vi "Read Key (Variant).vi"(5 "format string (%;%f)":string="%f", 7 "section":string, 8 "error in (no error)":errorcluster, 9 "type":variant, 10 "key (optional)":string, 11 "refnum":T1) -> (0 "error out":errorcluster, 1 "key-value":variant, 2 "found?":bool, 3 "refnum out":T1)   [LabVIEW 2020, in "openg_variant_configuration_file.lvlib"]
doc: "Reads a value associated with key in a specified section of the configuration data identified by refnum. If \"key\" input is not specified, the name of the variant object is used as the key. the \"found?\" output will be TRUE for compount objects (clusters) only if all elements (recursively) are found.\n\nFor example a Boolean named \"Enable\" with a value of TRUE would correspond to the key-value pair:\n\nEnable=TRUE\n\nNote: Special characters in section and key names will be escape-coded. These include the following: \\00-\\1F (non-printable chars); \"[\", \"]\", and \"=\" (INI syntax elements); \\FE (\"þ\") and \\FF (\"ÿ\") (legacy bracket encoding); Additionally, the escape character, \"\\\", will be escaped as \"\\\\\"."
uses:
  openg_variant_configuration_file.lvlib
  <vilib>/Utility/config.llb/Config Data RefNum.ctl
  <vilib>/Utility/config.llb/Read Key (I32).vi
  <vilib>/Utility/config.llb/Read Key (U32).vi
  <vilib>/Utility/config.llb/Read Key (Double).vi
  <vilib>/Utility/config.llb/Read Key (String).vi
  <vilib>/Utility/config.llb/Read Key (Boolean).vi
  <vilib>/Utility/config.llb/Read Key (Path).vi
  <vilib>/Utility/config.llb/NI_LVConfig.lvlib
  <userlib>/_OpenG.lib/lvdata/lvdata.llb/openg_variant.lvlib
panel:
  in  "Ref for recursive call":refnum<vi>
  # "Read Key (Variant).vi\n\nReads a variant key-value from INI file.\n\nPlease visit http://www.OpenG.org to learn about the\nOpen Source LabVIEW software movement.\n\nNOTICE -- YOU MUST LEAVE THIS NOTICE IN PLACE.  PER THE TERMS OF THE LICENSE BELOW, YOU MAY SUBLICENSE THIS SOFTWARE \nIN ANY WAY THAT DOES NOT CONFLICT WITH THIS LICENSE.\n\n### BSD License (http://www.opensource.org/licenses/bsd-license.php) Begin ###\n \nCopyright (c) 2002, Jean-Pierre Drolet <drolet_jp@hotmail.com>\nCopyright (c) 2002-2006, Jim Kring <jim@jimkring.com>\n\nAll rights reserved.\n\nRedistribution and use in source and binary forms, with or without modification, are permitted provided that the following conditions are met:\n\n    * Redistributions of source code must retain the above copyright notice, this list of conditions and the following disclaimer.\n    * Redistributions in binary form must reproduce the above copyright notice, this list of conditions and the following disclaimer in the \n       documentation and/or other materials provided with the distribution.\n    * Neither the name of SciWare, James Kring, Inc., nor the names of its contributors may be used to endorse or promote products derived \n       from this software without specific prior written permission.\n\nTHIS SOFTWARE IS PROVIDED BY THE COPYRIGHT HOLDERS AND CONTRIBUTORS \"AS IS\" AND ANY EXPRESS OR IMPLIED WARRANTIES, \nINCLUDING, BUT NOT LIMITED TO, THE IMPLIED WARRANTIES OF MERCHANTABILITY AND FITNESS FOR A PARTICULAR PURPOSE ARE \nDISCLAIMED. IN NO EVENT SHALL THE COPYRIGHT OWNER OR CONTRIBUTORS BE LIABLE FOR ANY DIRECT, INDIRECT, INCIDENTAL,\n SPECIAL, EXEMPLARY, OR CONSEQUENTIAL DAMAGES (INCLUDING, BUT NOT LIMITED TO, PROCUREMENT OF SUBSTITUTE GOODS OR \nSERVICES; LOSS OF USE, DATA, OR PROFITS; OR BUSINESS INTERRUPTION) HOWEVER CAUSED AND ON ANY THEORY OF LIABILITY, \nWHETHER IN CONTRACT, STRICT LIABILITY, OR TORT (INCLUDING NEGLIGENCE OR OTHERWISE) ARISING IN ANY WAY OUT OF THE USE \nOF THIS SOFTWARE, EVEN IF ADVISED OF THE POSSIBILITY OF SUCH DAMAGE.\n\n### BSD License End ###"
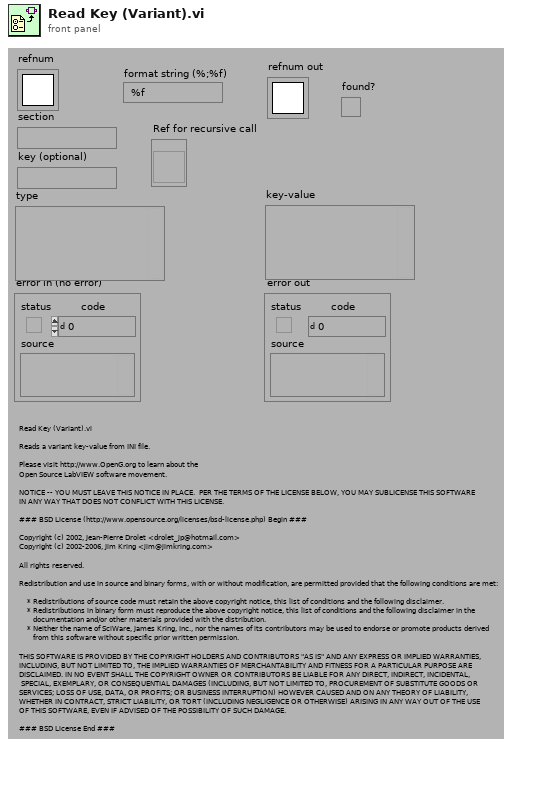
[diagram p1: front panel]
types:
  T1 = typedef "NI_LVConfig.lvlib/Config Data RefNum.ctl" = refnum<k1>
  T2 = typedef "openg_variant.lvlib/Type Descriptor Enumeration__ogtk.ctl" = enum8{"<Null>", "I8", "I16", "I32", "I64", "U8", "U16", "U32", "U64", "SGL", "DBL", "EXT", "CSG", "CDB", "CXT", "0x0F", "0x10", "0x11", "0x12", "0x13", "0x14", "Enum U8", "Enum U16", "Enum U32", "Enum U64", "SGL PQ", "DBL PQ", "EXT PQ", "CSG PQ", "CDB PQ", "CXT PQ", "0x1F", "0x20", "Boolean", "0x22", "0x23", "0x24", "0x25", "0x26", "0x27", "0x28", "0x29", "0x2A", "0x2B", "0x2C", "0x2D", "0x2E", "0x2F", "String", "0x31", "Path", "Pict", "0x34", "0x35", "0x36", "DAQ", "0x38", "0x39", "0x3A", "0x3B", "0x3C", "0x3D", "0x3E", "0x3F", "Array", "0x41", "0x42", "0x43", "0x44", "0x45", "0x46", "0x47", "0x48", "0x49", "0x4A", "0x4B", "0x4C", "0x4D", "0x4E", "0x4F", "Cluster", "0x51", "0x52", "Variant", "Waveform", "0x55", "0x56", "0x57", "0x58", "0x59", "0x5A", "0x5B", "0x5C", "0x5D", "0x5E", "Fixed Point", "0x60", "0x61", "0x62", "0x63", "0x64", "0x65", "0x66", "0x67", "0x68", "0x69", "0x6A", "0x6B", "0x6C", "0x6D", "0x6E", "0x6F", "Refnum", "0x71", "0x72", "Set Collection", "Map Collection"}
  T3 = typedef "openg_variant.lvlib/Type Descriptor__ogtk.ctl" = i16[]
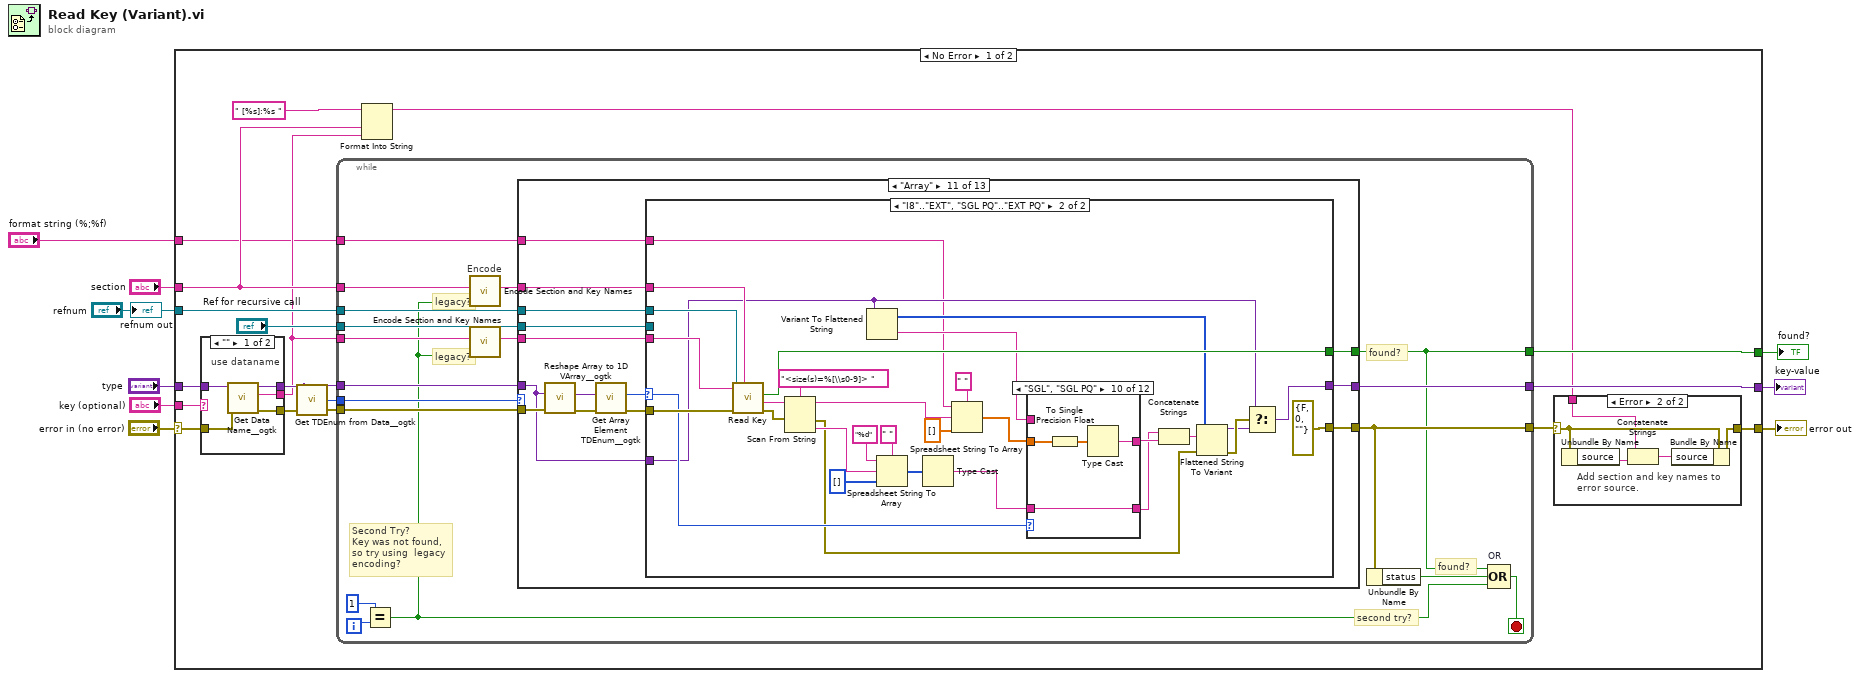
[diagram p0: block diagram]
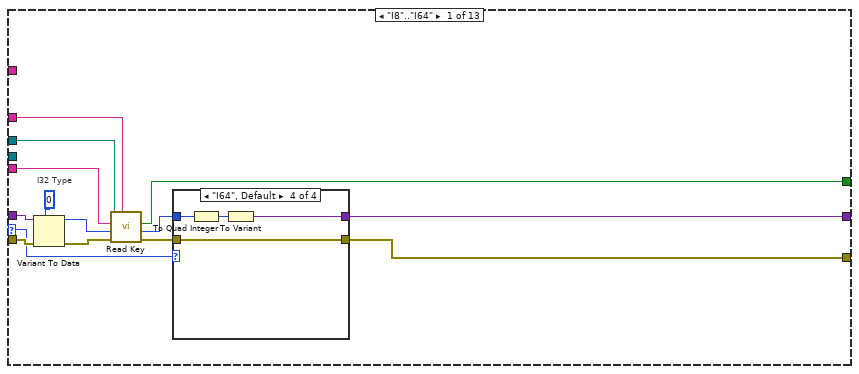
[diagram p2: hidden frame]
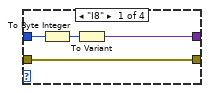
[diagram p3: hidden frame]
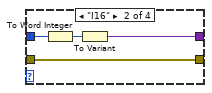
[diagram p4: hidden frame]
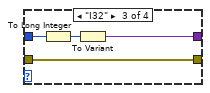
[diagram p5: hidden frame]
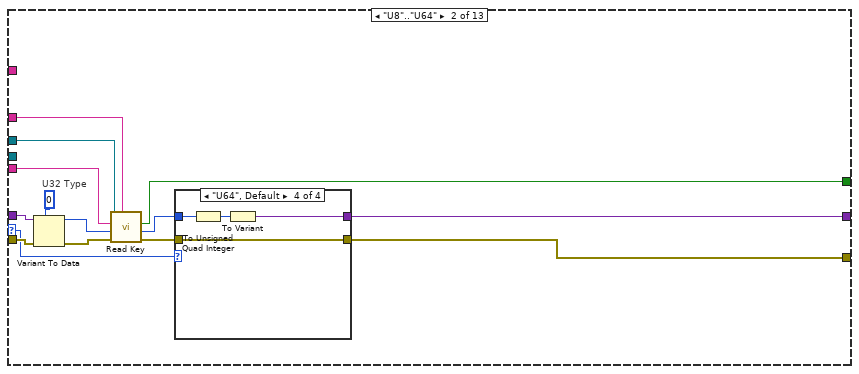
[diagram p6: hidden frame]
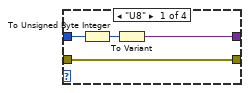
[diagram p7: hidden frame]
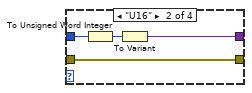
[diagram p8: hidden frame]
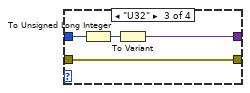
[diagram p9: hidden frame]
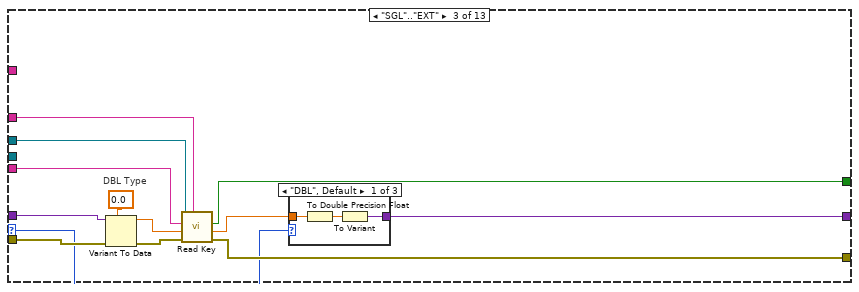
[diagram p10: hidden frame]
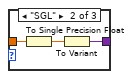
[diagram p11: hidden frame]
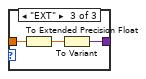
[diagram p12: hidden frame]
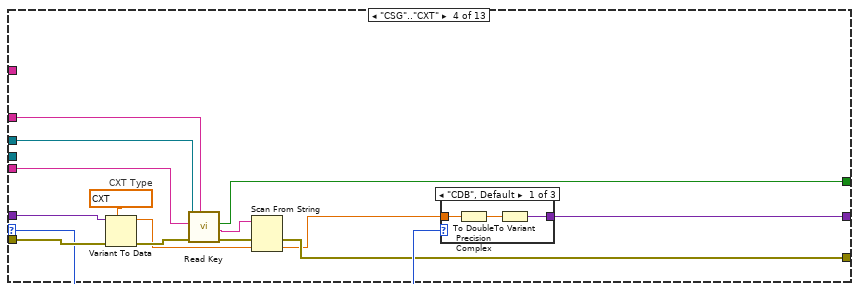
[diagram p13: hidden frame]
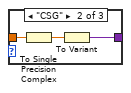
[diagram p14: hidden frame]
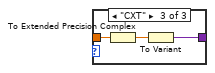
[diagram p15: hidden frame]
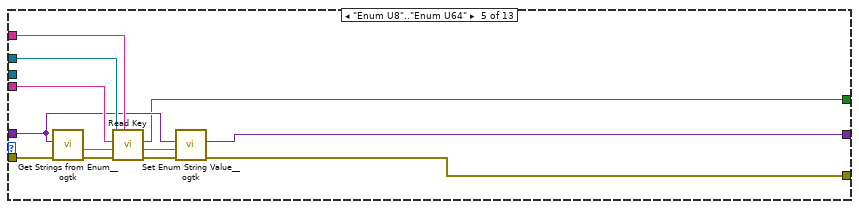
[diagram p16: hidden frame]
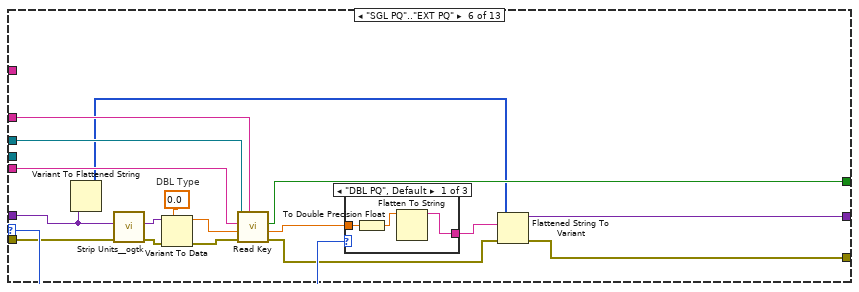
[diagram p17: hidden frame]
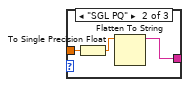
[diagram p18: hidden frame]
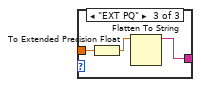
[diagram p19: hidden frame]
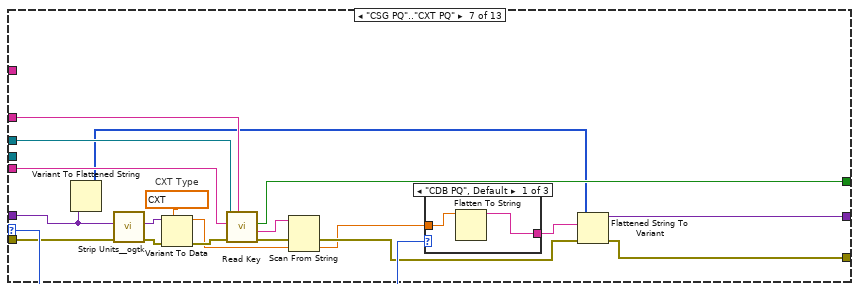
[diagram p20: hidden frame]
diagram:
  n1 = case shown="No Error" "error in (no error)" {
    selector: "error in (no error)" -> [w21 w480]
    tunnel: "refnum" -> [w25 _]
    tunnel: [w15 w480] -> w9
    tunnel: "type" -> [w23 _]
    tunnel: "key (optional)" -> [w22 _]
    tunnel: "section" -> [w12 _]
    tunnel: [w24 variant ("Variant")] -> w4
    tunnel: [w18 FALSE ("found?")] -> w2
    tunnel: "format string (%;%f)" -> [w10 _]
    frame No Error {
      n2 = case shown="\"\"" w22 {
        selector: w22 -> [_ w477]
        tunnel: [w474 w477] -> w11
        tunnel: w23 -> [w471 w475]
        tunnel: w21 -> [w473 w476]
        tunnel: [w472 w476] -> w20
        tunnel: [w470 w475] -> w19
        frame "" {
          # "use dataname"
          n3 = call <userlib>:"Get Data Name__ogtk.vi"("error in (no error)"=w473, "Data"=w471) -> ("error out"=w472:errorcluster, "Data Name"=w474:string, "Data dup"=w470:variant)  [unwired: 7 in]
        }
        frame Default {
          # "use optional\nkey"
        }
      }
      n4 = call <userlib>:"Get TDEnum from Data__ogtk.vi"("Data"=w19) -> ("Type Descriptor Enumeration"=w26:T2)  [unwired: 4 in]
      n5 = while {
        tunnel: w26 -> [w44]
        tunnel: w25 -> [w43]
        tunnel: [w42] -> w24
        tunnel: w20 -> [w41]
        tunnel: w19 -> [w40]
        tunnel: [w32] -> w18
        tunnel: "Ref for recursive call" -> [w39]
        tunnel: [w34] -> w16
        tunnel: w12 -> [w37]
        tunnel: w11 -> [w36]
        tunnel: w10 -> [w27]
        i -> [w31]
        stop <- w29 stop-if-true
        # "found?"
        # "found?"
        # "second try?"
        # "legacy?"
        # "legacy?"
        # "Second Try?\nKey was not found, so try using  legacy encoding?"
        # "Encode"
        n6 = Equal?(x=1, y=w31) -> (x = y?=w28:bool)
        n7 = call "Encode Section and Key Names.vi"("use legacy encoding scheme? (FALSE)"=w28, "string"=w37) -> ("encoded string"=w38:string)  [unwired: 9 in]
        n8 = call "Encode Section and Key Names.vi"("use legacy encoding scheme? (FALSE)"=w28, "string"=w36) -> ("encoded string"=w35:string)  [unwired: 9 in]
        n9 = case shown="\"Array\"" w44 {
          selector: w44 -> [w47 w77 w105 w132 _ w172 w203 _ _ _ _ _ _]
          tunnel: w40 -> [w57 w87 w116 w140 w153 w165 w197 w228 w240 w252 w256 w411 w460]
          tunnel: w43 -> [w56 w86 w115 w139 w162 w179 w208 w227 w239 w251 w263 w425 w463]
          tunnel: [w46 w75 w113 w130 w155 w167 w199 w225 w237 w249 w260 w414 w454] -> w34
          tunnel: w41 -> [w54 w84 w112 w137 w159 w171 w202 w224 w236 w248 w266 w413 w456]
          tunnel: w35 -> [w53 w83 w111 w136 w161 w177 w206 w223 w235 w247 w257 w423 w462]
          tunnel: w38 -> [w52 w82 w110 w135 w160 w176 w205 w222 w234 w246 w258 w424 w461]
          tunnel: [w45 w79 w107 w134 w152 w163 w195 w219 w233 w243 w261 w415 w457] -> w42
          tunnel: [w50 w78 w106 w133 w151 w173 w204 w218 w230 w242 w259 w419 w452] -> w32
          tunnel: w39 -> [_ _ _ _ _ _ _ _ _ _ w262 w418 _]
          tunnel: w27 -> [_ _ _ _ _ _ _ _ _ _ w254 w408 _]
          frame "I8".."I64" {
            # "I32 Type"
            n10 = Variant To Data(error in=w54, type=0, Variant=w57) -> (data=w51:i32, error out=w55:errorcluster)
            n11 = call-poly <vilib>:"Read Key.vi"("section"=w52, "error in (no error)"=w55, "default value"=w51, "key"=w53, "refnum"=w56) -> ("error out"=w49:errorcluster, "value"=w48:i32, "found?"=w50:bool)  [unwired: 3 in, 1 out]
            n12 = case shown="\"I64\", Default" w47 {
              tunnel: w48 -> [w62 w66 w70 w74]
              tunnel: [w61 w65 w69 w73] -> w45
              tunnel: w49 -> [w59 w63 w67 w71]
              tunnel: [w59 w63 w67 w71] -> w46
              frame "I8" {
                n13 = To Byte Integer(number=w62) -> (8bit integer=w60:i8)
                n14 = To Variant(anything=w60) -> (Variant=w61:variant)
              }
              frame "I16" {
                n15 = To Word Integer(number=w66) -> (16bit integer=w64:i16)
                n16 = To Variant(anything=w64) -> (Variant=w65:variant)
              }
              frame "I32" {
                n17 = To Long Integer(number=w70) -> (32bit integer=w68:i32)
                n18 = To Variant(anything=w68) -> (Variant=w69:variant)
              }
              frame "I64", Default {
                n19 = To Quad Integer(1:w74) -> (0:w72:i64)
                n20 = To Variant(anything=w72) -> (Variant=w73:variant)
              }
            }
          }
          frame "U8".."U64" {
            # "U32 Type"
            n21 = Variant To Data(error in=w84, type=u32 0, Variant=w87) -> (data=w81:u32, error out=w85:errorcluster)
            n22 = call-poly <vilib>:"Read Key.vi"("section"=w82, "error in (no error)"=w85, "default value"=w81, "key"=w83, "refnum"=w86) -> ("error out"=w76:errorcluster, "value"=w80:u32, "found?"=w78:bool)  [unwired: 3 in, 1 out]
            n23 = case shown="\"U64\", Default" w77 {
              tunnel: w80 -> [w92 w96 w100 w104]
              tunnel: [w91 w95 w99 w103] -> w79
              tunnel: w76 -> [w89 w93 w97 w101]
              tunnel: [w89 w93 w97 w101] -> w75
              frame "U8" {
                n24 = To Unsigned Byte Integer(number=w92) -> (unsigned 8bit integer=w90:u8)
                n25 = To Variant(anything=w90) -> (Variant=w91:variant)
              }
              frame "U16" {
                n26 = To Unsigned Word Integer(number=w96) -> (unsigned 16bit integer=w94:u16)
                n27 = To Variant(anything=w94) -> (Variant=w95:variant)
              }
              frame "U32" {
                n28 = To Unsigned Long Integer(number=w100) -> (unsigned 32bit integer=w98:u32)
                n29 = To Variant(anything=w98) -> (Variant=w99:variant)
              }
              frame "U64", Default {
                n30 = To Unsigned Quad Integer(1:w104) -> (0:w102:u64)
                n31 = To Variant(anything=w102) -> (Variant=w103:variant)
              }
            }
          }
          frame "SGL".."EXT" {
            # "DBL Type"
            n32 = Variant To Data(error in=w112, type=0.0, Variant=w116) -> (data=w109:dbl, error out=w114:errorcluster)
            n33 = call-poly <vilib>:"Read Key.vi"("section"=w110, "error in (no error)"=w114, "default value"=w109, "key"=w111, "refnum"=w115) -> ("error out"=w113:errorcluster, "value"=w108:dbl, "found?"=w106:bool)  [unwired: 3 in, 1 out]
            n34 = case shown="\"DBL\", Default" w105 {
              tunnel: w108 -> [w120 w123 w126]
              tunnel: [w119 w122 w125] -> w107
              frame "DBL", Default {
                n35 = To Double Precision Float(number=w120) -> (double precision float=w118:dbl)
                n36 = To Variant(anything=w118) -> (Variant=w119:variant)
              }
              frame "SGL" {
                n37 = To Single Precision Float(number=w123) -> (single precision float=w121:sgl)
                n38 = To Variant(anything=w121) -> (Variant=w122:variant)
              }
              frame "EXT" {
                n39 = To Extended Precision Float(1:w126) -> (0:w124:ext)
                n40 = To Variant(anything=w124) -> (Variant=w125:variant)
              }
            }
          }
          frame "CSG".."CXT" {
            # "CXT Type"
            n41 = Variant To Data(error in=w137, type=cxt 0.0+0.0i, Variant=w140) -> (data=w128:cxt, error out=w138:errorcluster)
            n42 = call-poly <vilib>:"Read Key.vi"("section"=w135, "error in (no error)"=w138, "key"=w136, "refnum"=w139) -> ("error out"=w131:errorcluster, "value"=w129:string, "found?"=w133:bool)  [unwired: 4 in, 1 out]
            n43 = Scan From String(input string=w129, error in=w131, default 1=w128) -> (error out=w130:errorcluster, output 1=w127:cxt)  [unwired: 2 in, 2 out]
            n44 = case shown="\"CDB\", Default" w132 {
              tunnel: w127 -> [w144 w147 w150]
              tunnel: [w143 w146 w149] -> w134
              frame "CDB", Default {
                n45 = To Double Precision Complex(1:w144) -> (0:w142:cdb)
                n46 = To Variant(anything=w142) -> (Variant=w143:variant)
              }
              frame "CSG" {
                n47 = To Single Precision Complex(1:w147) -> (0:w145:csg)
                n48 = To Variant(anything=w145) -> (Variant=w146:variant)
              }
              frame "CXT" {
                n49 = To Extended Precision Complex(1:w150) -> (0:w148:cxt)
                n50 = To Variant(anything=w148) -> (Variant=w149:variant)
              }
            }
          }
          frame "Enum U8".."Enum U64" {
            n51 = call <userlib>:"Get Strings from Enum__ogtk.vi"("error in (no error)"=w159, "Enum"=w153) -> ("error out"=w158:errorcluster, "String Value"=w157:string)  [unwired: 6 in, 2 out]
            n52 = call-poly <vilib>:"Read Key.vi"("section"=w160, "error in (no error)"=w158, "default value"=w157, "key"=w161, "refnum"=w162) -> ("error out"=w156:errorcluster, "value"=w154:string, "found?"=w151:bool)  [unwired: 3 in, 1 out]
            n53 = call <userlib>:"Set Enum String Value__ogtk.vi"("error in (no error)"=w156, "String Value"=w154, "Default Enum Value"=w153) -> ("error out"=w155:errorcluster, "Enum"=w152:variant)  [unwired: 7 in]
          }
          frame "SGL PQ".."EXT PQ" {
            # "DBL Type"
            n54 = Variant To Flattened String(Variant=w165) -> (1:w164:i16[])  [unwired: 1 out]
            n55 = call <userlib>:"Strip Units__ogtk.vi"("error in (no error)"=w171, "Number or 1D array with units"=w165) -> ("error out"=w169:errorcluster, "Pure Number(s) (base units)"=w170:variant)  [unwired: 8 in]
            n56 = Variant To Data(error in=w169, type=0.0, Variant=w170) -> (data=w175:dbl, error out=w178:errorcluster)
            n57 = call-poly <vilib>:"Read Key.vi"("section"=w176, "error in (no error)"=w178, "default value"=w175, "key"=w177, "refnum"=w179) -> ("error out"=w168:errorcluster, "value"=w174:dbl, "found?"=w173:bool)  [unwired: 3 in, 1 out]
            n58 = case shown="\"DBL PQ\", Default" w172 {
              tunnel: w174 -> [w183 w186 w189]
              tunnel: [w182 w184 w187] -> w166
              frame "DBL PQ", Default {
                n59 = To Double Precision Float(number=w183) -> (double precision float=w181:dbl)
                n60 = Flatten To String(anything=w181) -> (data string=w182:string)  [unwired: 3 in, 2 out]
              }
              frame "SGL PQ" {
                n61 = To Single Precision Float(number=w186) -> (single precision float=w185:sgl)
                n62 = Flatten To String(anything=w185) -> (data string=w184:string)  [unwired: 3 in, 2 out]
              }
              frame "EXT PQ" {
                n63 = To Extended Precision Float(1:w189) -> (0:w188:ext)
                n64 = Flatten To String(anything=w188) -> (data string=w187:string)  [unwired: 3 in, 2 out]
              }
            }
            n65 = Flattened String To Variant(4:w168, 6:w166, 7:w164) -> (0:w167:errorcluster, 3:w163:variant)
          }
          frame "CSG PQ".."CXT PQ" {
            # "CXT Type"
            n66 = Variant To Flattened String(Variant=w197) -> (1:w196:i16[])  [unwired: 1 out]
            n67 = call <userlib>:"Strip Units__ogtk.vi"("error in (no error)"=w202, "Number or 1D array with units"=w197) -> ("error out"=w200:errorcluster, "Pure Number(s) (base units)"=w201:variant)  [unwired: 8 in]
            n68 = Variant To Data(error in=w200, type=cxt 0.0+0.0i, Variant=w201) -> (data=w191:cxt, error out=w207:errorcluster)
            n69 = call-poly <vilib>:"Read Key.vi"("section"=w205, "error in (no error)"=w207, "key"=w206, "refnum"=w208) -> ("error out"=w193:errorcluster, "value"=w192:string, "found?"=w204:bool)  [unwired: 4 in, 1 out]
            n70 = Scan From String(input string=w192, error in=w193, default 1=w191) -> (error out=w194:errorcluster, output 1=w190:cxt)  [unwired: 2 in, 2 out]
            n71 = case shown="\"CDB PQ\", Default" w203 {
              tunnel: w190 -> [w211 w214 w217]
              tunnel: [w210 w212 w215] -> w198
              frame "CDB PQ", Default {
                n72 = Flatten To String(anything=w211) -> (data string=w210:string)  [unwired: 3 in, 2 out]
              }
              frame "CSG PQ" {
                n73 = To Single Precision Complex(1:w214) -> (0:w213:csg)
                n74 = Flatten To String(anything=w213) -> (data string=w212:string)  [unwired: 3 in, 2 out]
              }
              frame "CXT PQ" {
                n75 = To Extended Precision Complex(1:w217) -> (0:w216:cxt)
                n76 = Flatten To String(anything=w216) -> (data string=w215:string)  [unwired: 3 in, 2 out]
              }
            }
            n77 = Flattened String To Variant(4:w194, 6:w198, 7:w196) -> (0:w199:errorcluster, 3:w195:variant)
          }
          frame "Boolean" {
            # "Boolean Type"
            n78 = Variant To Data(error in=w224, type=FALSE, Variant=w228) -> (data=w221:bool, error out=w226:errorcluster)
            n79 = call-poly <vilib>:"Read Key.vi"("section"=w222, "error in (no error)"=w226, "default value"=w221, "key"=w223, "refnum"=w227) -> ("error out"=w225:errorcluster, "value"=w220:bool, "found?"=w218:bool)  [unwired: 3 in, 1 out]
            n80 = To Variant(anything=w220) -> (Variant=w219:variant)
          }
          frame "String", "DAQ" {
            # "String Type"
            n81 = Variant To Data(error in=w236, type="", Variant=w240) -> (data=w231:string, error out=w238:errorcluster)
            n82 = call-poly <vilib>:"Read Key.vi"("section"=w234, "error in (no error)"=w238, "default value"=w231, "key"=w235, "refnum"=w239) -> ("error out"=w237:errorcluster, "value"=w232:string, "found?"=w230:bool)  [unwired: 3 in, 1 out]
            n83 = To Variant(anything=w232) -> (Variant=w233:variant)
          }
          frame "Path" {
            # "Path Type"
            n84 = Variant To Data(error in=w248, type=path "", Variant=w252) -> (data=w245:path, error out=w250:errorcluster)
            n85 = call-poly <vilib>:"Read Key.vi"("section"=w246, "error in (no error)"=w250, "default value"=w245, "key"=w247, "refnum"=w251) -> ("error out"=w249:errorcluster, "value"=w244:path, "found?"=w242:bool)  [unwired: 3 in, 1 out]
            n86 = To Variant(anything=w244) -> (Variant=w243:variant)
          }
          frame "Array" {
            n87 = call <userlib>:"Reshape Array to 1D VArray__ogtk.vi"("error in (no error)"=w266, "MultiD Array"=w256) -> ("error out"=w267:errorcluster, "1D VArray"=w255:variant)  [unwired: 7 in, 1 out]
            n88 = call <userlib>:"Get Array Element TDEnum__ogtk.vi"("error in (no error)"=w267, "Array"=w255) -> ("error out"=w264:errorcluster, "Element Type"=w265:T2)  [unwired: 8 in]
            n89 = case shown="\"I8\"..\"EXT\", \"SGL PQ\"..\"EXT PQ\"" w265 {
              selector: w265 -> [_ w346]
              tunnel: w264 -> [_ w356]
              tunnel: w256 -> [w277 w334]
              tunnel: w258 -> [w275 w357]
              tunnel: w263 -> [w274 w358]
              tunnel: w257 -> [w278 w359]
              tunnel: w262 -> [w276 _]
              tunnel: [w272 w333] -> w261
              tunnel: [w271 errorcluster {"status"=FALSE, "code"=0, "source"=""} ("error out")] -> w260
              tunnel: [w270 w355] -> w259
              tunnel: w254 -> [w268 w331]
              frame Default {
                n90 = Concatenate Strings(w278, ".<size(s)>" ("Substring")) -> (w281:string)
                n91 = call-poly <vilib>:"Read Key.vi"("read raw string? (F)"=TRUE, "section"=w275, "key"=w281, "refnum"=w274) -> ("error out"=w279:errorcluster, "value"=w280:string, "found?"=w269:bool)  [unwired: 4 in, 1 out]
                n92 = case shown="True" w269 {
                  tunnel: w280 -> [_ w312]
                  tunnel: w279 -> [_ w288]
                  tunnel: w278 -> [_ w307]
                  tunnel: w277 -> [w284 w306]
                  tunnel: w276 -> [_ w305]
                  tunnel: w275 -> [_ w303]
                  tunnel: w274 -> [_ w302]
                  tunnel: [w284 w295] -> w272
                  tunnel: [errorcluster {"status"=FALSE, "code"=0, "source"=""} ("error out") w294] -> w271
                  tunnel: [FALSE w292] -> w270
                  tunnel: w268 -> [_ w286]
                  frame False {
                    # "array size(s) not found. Ignore element keys (if any) and return input array"
                  }
                  frame True {
                    # "array.size(s) is found. Read elements keys. missing keys replace with datatype default."
                    n93 = call <userlib>:"Get Array Element TD__ogtk.vi"("error in (no error)"=w288, "Array"=w306) -> ("error out"=w290:errorcluster, "Type Descriptor"=w291:T3)  [unwired: 8 in]
                    n94 = property class="VI"() -> ("VI Name"=w309:string)  [unwired: 2 in, 2 out]
                    n95 = call <userlib>:"Get Default Data from TD__ogtk.vi"("error in (no error)"=w290, "Type Descriptor"=w291) -> ("error out"=w287:errorcluster, "Default VData"=w289:variant)  [unwired: 8 in]
                    n96 = Spreadsheet String To Array(delimiter (Tab)=" ", format string="%d", spreadsheet string=w312, array type (2D Dbl)=u32[] [] ("Array Constant")) -> (array=w296:u32[])
                    n97 = Open VI Reference(type specifier VI Refnum (for type only)=w305, vi path=w309, error in (no error)=w287) -> (vi reference=w304:refnum<vi>, error out=w308:errorcluster)  [unwired: 3 in]
                    n98 = Multiply Array Elements(1:w296) -> (0:w310:u32)
                    n99 = for {
                      N: w310 -> [_]
                      shift-right: [w324] -> w299
                      shift-left: w308 -> [w321]
                      shift-right: [w325] -> w301
                      shift-left: w304 -> [w323]
                      tunnel: w307 -> [w328]
                      tunnel: w289 -> [w322]
                      tunnel: w303 -> [w319]
                      tunnel: w302 -> [w318]
                      tunnel: [w317] -> w300 mode=indexing
                      tunnel: [w316] -> w293 mode=indexing
                      tunnel: w286 -> [w315]
                      i -> [w329]
                      n100 = Format Into String(format string=" %d" ("Format String"), initial string=w328, w329) -> (resulting string=w320:string)  [unwired: 1 in, 1 out]
                      n101 = call-by-ref "?"(reference=w323, error in=w321, "format string (%;%f"=w315, "section"=w319, "type"=w322, "key (optional)"=w320, "refnum"=w318) -> (reference out=w325:refnum<vi>, error out=w327:errorcluster, "error out"=w326:errorcluster, "key-value"=w317:variant, "found?"=w316:bool)  [unwired: 3 in, 1 out]
                      n102 = Merge Errors(w327, w326) -> (w324:errorcluster)
                    }
                    n103 = And Array Elements(Boolean array=w293) -> (logical AND=w292:bool)
                    n104 = Close Reference(reference=w301) -> ()  [unwired: 1 in, 1 out]
                    n105 = call <userlib>:"Array of VData to VArray__ogtk.vi"("error in (no error)"=w299, "Element Type (when empty)"=w289, "1D Array of VData"=w300) -> ("error out"=w298:errorcluster, "VArray"=w297:variant)  [unwired: 7 in]
                    n106 = call <userlib>:"Reshape 1D Array__ogtk.vi"("error in (no error)"=w298, "Size(s)"=w296, "1D Array"=w297) -> ("error out"=w294:errorcluster, "Reshaped VArray"=w295:variant)  [unwired: 7 in]
                  }
                }
              }
              frame "I8".."EXT", "SGL PQ".."EXT PQ" {
                n107 = call-poly <vilib>:"Read Key.vi"("section"=w357, "error in (no error)"=w356, "key"=w359, "refnum"=w358) -> ("error out"=w354:errorcluster, "value"=w360:string, "found?"=w355:bool)  [unwired: 4 in, 1 out]
                n108 = Scan From String(format string="<size(s)=%[\\s0-9]> " ("regular expression"), input string=w360, error in=w354) -> (remaining string=w347:string, error out=w337:errorcluster, output 1=w352:string)  [unwired: 2 in, 1 out]
                n109 = Variant To Flattened String(Variant=w334) -> (data string=w339:string, 1:w340:i16[])
                n110 = Spreadsheet String To Array(delimiter (Tab)=" ", format string="%d", spreadsheet string=w352, array type (2D Dbl)=u32[] []) -> (array=w353:u32[])
                n111 = Type Cast(x=w353) -> (*(type *) &x=w344:string)  [unwired: 1 in]
                n112 = Spreadsheet String To Array(delimiter (Tab)=" ", format string=w331, spreadsheet string=w347, array type (2D Dbl)=dbl[] []) -> (array=w345:dbl[])
                n113 = case shown="\"SGL\", \"SGL PQ\"" w346 {
                  tunnel: w345 -> [_ w367 w371 w375 w379 w383 w387 w391 w395 w399 w401 w405]
                  tunnel: [w362 w365 w369 w373 w377 w381 w385 w389 w393 w397 w403 w407] -> w342
                  tunnel: ["" w364 w368 w372 w376 w380 w384 w388 w392 w396 w402 w406] -> w341
                  tunnel: w344 -> [_ w364 w368 w372 w376 w380 w384 w388 w392 w396 w402 w406]
                  tunnel: w339 -> [w362 _ _ _ _ _ _ _ _ _ _ _]
                  frame Default {
                  }
                  frame "I8" {
                    n114 = To Byte Integer(number=w367) -> (8bit integer=w366:i8[])
                    n115 = Type Cast(x=w366) -> (*(type *) &x=w365:string)  [unwired: 1 in]
                  }
                  frame "I16" {
                    n116 = To Word Integer(number=w371) -> (16bit integer=w370:i16[])
                    n117 = Type Cast(x=w370) -> (*(type *) &x=w369:string)  [unwired: 1 in]
                  }
                  frame "I32" {
                    n118 = To Long Integer(number=w375) -> (32bit integer=w374:i32[])
                    n119 = Type Cast(x=w374) -> (*(type *) &x=w373:string)  [unwired: 1 in]
                  }
                  frame "I64" {
                    n120 = To Quad Integer(1:w379) -> (0:w378:i64[])
                    n121 = Type Cast(x=w378) -> (*(type *) &x=w377:string)  [unwired: 1 in]
                  }
                  frame "U8" {
                    n122 = To Unsigned Byte Integer(number=w383) -> (unsigned 8bit integer=w382:u8[])
                    n123 = Type Cast(x=w382) -> (*(type *) &x=w381:string)  [unwired: 1 in]
                  }
                  frame "U16" {
                    n124 = To Unsigned Word Integer(number=w387) -> (unsigned 16bit integer=w386:u16[])
                    n125 = Type Cast(x=w386) -> (*(type *) &x=w385:string)  [unwired: 1 in]
                  }
                  frame "U32" {
                    n126 = To Unsigned Long Integer(number=w391) -> (unsigned 32bit integer=w390:u32[])
                    n127 = Type Cast(x=w390) -> (*(type *) &x=w389:string)  [unwired: 1 in]
                  }
                  frame "U64" {
                    n128 = To Unsigned Quad Integer(1:w395) -> (0:w394:u64[])
                    n129 = Type Cast(x=w394) -> (*(type *) &x=w393:string)  [unwired: 1 in]
                  }
                  frame "SGL", "SGL PQ" {
                    n130 = To Single Precision Float(number=w399) -> (single precision float=w398:sgl[])
                    n131 = Type Cast(x=w398) -> (*(type *) &x=w397:string)  [unwired: 1 in]
                  }
                  frame "DBL", "DBL PQ" {
                    n132 = To Double Precision Float(number=w401) -> (double precision float=w400:dbl[])
                    n133 = Type Cast(x=w400) -> (*(type *) &x=w403:string)  [unwired: 1 in]
                  }
                  frame "EXT", "EXT PQ" {
                    n134 = To Extended Precision Float(1:w405) -> (0:w404:ext[])
                    n135 = Type Cast(x=w404) -> (*(type *) &x=w407:string)  [unwired: 1 in]
                  }
                }
                n136 = Concatenate Strings(w341, w342) -> (w343:string)
                n137 = Flattened String To Variant(4:w337, 6:w343, 7:w340) -> (0:w336:errorcluster, 3:w335:variant)
                n138 = Select(t=w334, s=w336, f=w335) -> (s? t:f=w333:variant)
              }
            }
          }
          frame "Cluster" {
            # ">> Cluster Name >>"
            # "Expand cluster to its elements\nand read keys recursively."
            n139 = call <userlib>:"Get Data Name__ogtk.vi"("error in (no error)"=w413, "Data"=w411) -> ("error out"=w412:errorcluster, "Data Name"=w409:string, "Data dup"=w410:variant)  [unwired: 7 in]
            n140 = call <userlib>:"Cluster to Array of VData__ogtk.vi"("error in (no error)"=w412, "Cluster"=w410) -> ("error out"=w431:errorcluster, "Array of VData"=w430:variant[])  [unwired: 8 in]
            n141 = property class="VI"() -> ("VI Name"=w429:string)  [unwired: 2 in, 2 out]
            n142 = Open VI Reference(type specifier VI Refnum (for type only)=w418, vi path=w429, error in (no error)=w431) -> (vi reference=w426:refnum<vi>, error out=w428:errorcluster)  [unwired: 3 in]
            n143 = for {
              shift-right: [w450] -> w427
              shift-left: w426 -> [w451]
              shift-right: [w435] -> w421
              shift-left: w428 -> [w446]
              tunnel: w430 -> [w444] mode=indexing
              tunnel: w424 -> [w440]
              tunnel: w425 -> [w441]
              tunnel: w423 -> [w448]
              tunnel: [w437] -> w422 mode=indexing
              tunnel: [w433] -> w420 mode=indexing
              tunnel: w408 -> [w432]
              n144 = call <userlib>:"Get Data Name__ogtk.vi"("error in (no error)"=w446, "Data"=w444) -> ("error out"=w445:errorcluster, "Data Name"=w434:string, "Data dup"=w443:variant)  [unwired: 7 in]
              n145 = Format Into String(format string=".%s" ("Format String"), initial string=w448, w434) -> (resulting string=w442:string)  [unwired: 1 in, 1 out]
              n146 = call-by-ref "?"(reference=w451, error in=w445, "format string (%;%f"=w432, "section"=w440, "type"=w443, "key (optional)"=w442, "refnum"=w441) -> (reference out=w450:refnum<vi>, error out=w449:errorcluster, "error out"=w439:errorcluster, "key-value"=w438:variant, "found?"=w433:bool)  [unwired: 3 in, 1 out]
              n147 = Merge Errors(w449, w439) -> (w436:errorcluster)
              n148 = call <userlib>:"Set Data Name__ogtk.vi"("error in (no error)"=w436, "Data Name"=w434, "Data"=w438) -> ("error out"=w435:errorcluster, "Renamed Data"=w437:variant)  [unwired: 7 in]
            }
            n149 = And Array Elements(Boolean array=w420) -> (logical AND=w419:bool)
            n150 = call <userlib>:"Array of VData to VCluster__ogtk.vi"("error in (no error)"=w421, "Array"=w422) -> ("error out"=w417:errorcluster, "VCluster"=w416:variant)  [unwired: 8 in]
            n151 = Close Reference(reference=w427) -> ()  [unwired: 1 in, 1 out]
            n152 = call <userlib>:"Set Data Name__ogtk.vi"("error in (no error)"=w417, "Data Name"=w409, "Data"=w416) -> ("error out"=w414:errorcluster, "Renamed Data"=w415:variant)  [unwired: 7 in]
          }
          frame Default {
            n153 = Variant To Flattened String(Variant=w460) -> (data string=w459:string, 1:w453:i16[])
            n154 = call-poly <vilib>:"Read Key.vi"("section"=w461, "error in (no error)"=w456, "default value"=w459, "key"=w462, "refnum"=w463) -> ("error out"=w455:errorcluster, "value"=w458:string, "found?"=w452:bool)  [unwired: 3 in, 1 out]
            n155 = Flattened String To Variant(4:w455, 6:w458, 7:w453) -> (0:w454:errorcluster, 3:w457:variant)
          }
        }
        n156 = Unbundle By Name(w34) -> ("status"=w33:bool)
        n157 = Compound Arithmetic op=OR "OR"(w32, w33, w28) -> (w29:bool)
      }
      n158 = Format Into String(format string=" [%s]:%s " ("Format String"), w12, w11) -> (resulting string=w13:string)  [unwired: 2 in, 1 out]
      n159 = case shown="Error" w16 {
        selector: w16 -> [w464 w469]
        tunnel: [w464 w468] -> w15
        tunnel: w13 -> [_ w465]
        frame No Error {
        }
        frame Error {
          # "Add section and key names to\nerror source."
          n160 = Unbundle By Name(w469) -> ("source"=w466:string)
          n161 = Concatenate Strings(w465, w466) -> (w467:string)
          n162 = Bundle By Name(cluster=w469, "source"=w467) -> (w468:errorcluster)
        }
      }
    }
    frame Error {
    }
  }
  "error out" <- w9
  "key-value" <- w4
  "found?" <- w2
  "refnum out" <- "refnum"
